vi "test Scheduled Loopback Value Overflow.vi"(8 "error in":errorcluster, 11 "TestCase in":refnum<class "Octal Loopback.lvclass">) -> (0 "error out":errorcluster, 3 "TestCase out":refnum<class "Octal Loopback.lvclass">)   [LabVIEW 2020, in "Octal Loopback.lvclass"]
uses:
  Octal Loopback.lvclass
  C:/Program Files (x86)/National Instruments/LabVIEW 2020/vi.lib/NI/VeriStand Custom Device Testing Tools/VeriStandTestCase/VeriStandTestCase.lvclass
  <vilib>/numeric/Random Number (Range) U64.vi
  <vilib>/numeric/sub_Random U32.vi
  <vilib>/NI VeriStand/Execution/Workspace/NI VeriStand - Set Multiple Channel Values.vi
  <vilib>/addons/_JKI Toolkits/VI Tester/TestCase.llb/TestCase.lvclass
  <vilib>/NI VeriStand/Execution/Workspace/NI_VS Workspace ExecutionAPI.lvlib
  <vilib>/NI/VeriStand Custom Device Testing Tools/VeriStandTestUtilities/VeriStandTestUtilities.lvlib
  C:/Program Files (x86)/National Instruments/LabVIEW 2020/vi.lib/addons/_JKI Toolkits/VI Tester/TestCase.llb/TestCase.lvclass
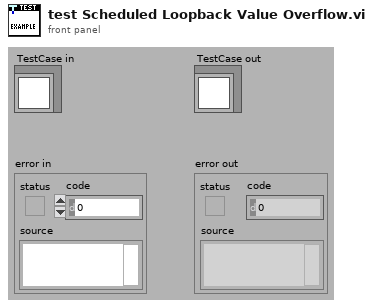
[diagram p1: front panel]
types:
  T1 = typedef "NI_VS Workspace ExecutionAPI.lvlib/WorkspaceAPI.ctl" = refnum<k24>
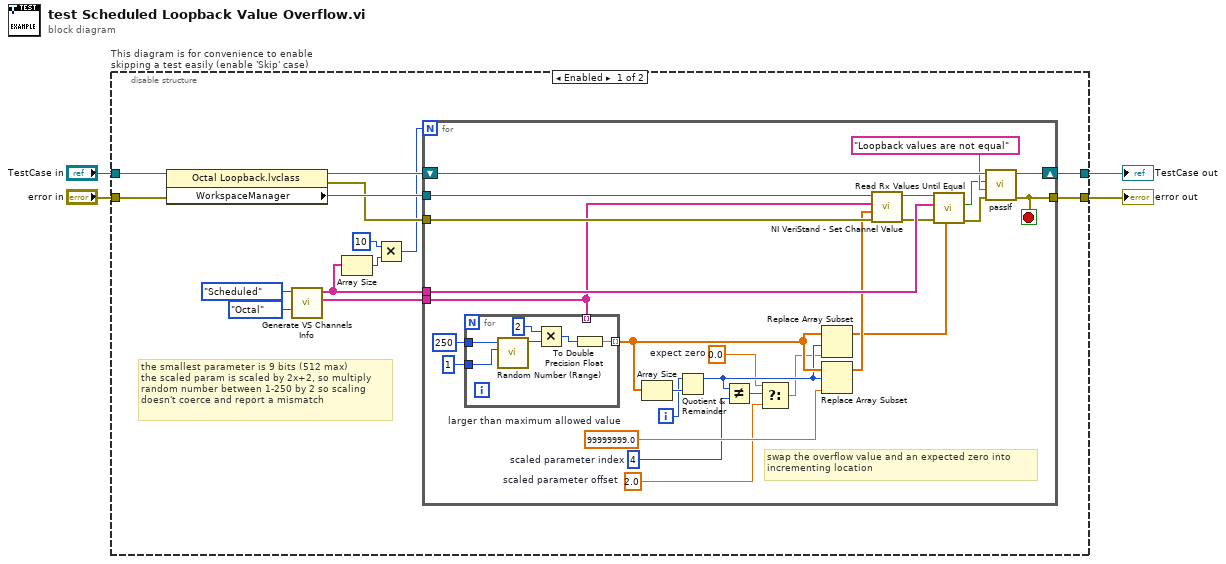
[diagram p0: block diagram]
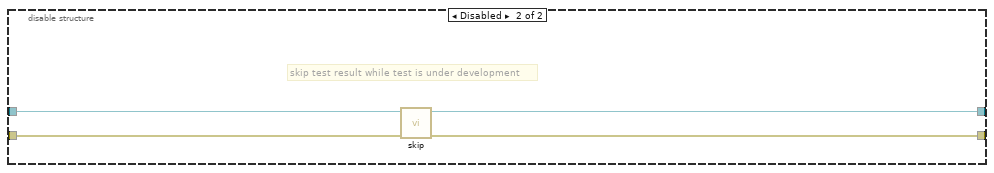
[diagram p2: hidden frame]
diagram:
  n1 = disable-structure "This diagram is for convenience to enable skipping a test easily (enable 'Skip' case)" shown="Enabled" {
    disable-tunnel: "TestCase in" -> [w15 w54]
    disable-tunnel: [w13 w52] -> w1
    disable-tunnel: [w12 w53] -> w3
    disable-tunnel: "error in" -> [w14 w51]
    frame Enabled {
      # "the smallest parameter is 9 bits (512 max)\nthe scaled param is scaled by 2x+2, so multiply \nrandom number between 1-250 by 2 so scaling\ndoesn't coerce and report a mismatch"
      n2 = property class="Octal Loopback.lvclass"(reference=w15, error in=w14) -> (reference out=w16:refnum<class "Octal Loopback.lvclass">, error out=w17:errorcluster, "WorkspaceManager"=w18:T1)
      n3 = call "Generate VS Channels Info.vi"("Label Format (Decimal)"=enum16{"Decimal", "Octal"}."Octal", "Transfer Type"=enum16{"Acyclic", "Scheduled"}."Scheduled") -> ("Tx Channels Array"=w11:string[], "Rx Channels Array"=w10:string[])  [unwired: 5 in, 3 out]
      n4 = Array Size(array=w10) -> (size(s)=w9:i32)
      n5 = Multiply(x=10, y=w9) -> (x*y=w7:i32)
      n6 = for {
        N: w7 -> [_]
        tunnel: w10 -> [w37]
        tunnel: w18 -> [w31]
        tunnel: w17 -> [w36]
        tunnel: w11 -> [w30]
        shift-right: [w43] -> w13
        shift-left: w16 -> [w44]
        tunnel: [w42] -> w12
        i -> [w25]
        stop <- w42 stop-if-true
        w20 = 2.0  # scaled parameter offset
        w23 = 4  # scaled parameter index
        w21 = 0.0  # expect zero
        w38 = 99999999.0  # larger than maximum allowed value
        # "swap the overflow value and an expected zero into \nincrementing location"
        n7 = for {
          tunnel: [w49] -> w26 mode=indexing
          tunnel: u64 250 ("upper bound (100)") -> [w48]
          tunnel: u64 1 ("upper bound (100)") -> [w47]
          tunnel: w30 -> [_] mode=indexing
          n8 = call-poly <vilib>:"Random Number (Range).vi"("lower bound (0)"=w47, "upper bound (100)"=w48) -> ("number"=w50:u64)  [unwired: 9 in]
          n9 = Multiply(x=u64 2, y=w50) -> (x*y=w46:u64)
          n10 = To Double Precision Float(number=w46) -> (double precision float=w49:dbl)
        }
        n11 = Array Size(array=w26) -> (size(s)=w27:i32)
        n12 = Quotient & Remainder(x=w25, y=w27) -> (x-y*floor(x/y)=w24:i32)  [unwired: 1 out]
        n13 = Not Equal?(x=w24, y=w23) -> (x != y?=w22:bool)
        n14 = Select(t=w21, s=w22, f=w20) -> (s? t:f=w19:dbl)
        n15 = Replace Array Subset(array=w26, new element=w19, index=w24) -> (w28:dbl[])
        n16 = Replace Array Subset(array=w26, new element=w38, index=w24) -> (w29:dbl[])
        n17 = call-poly <vilib>:"NI VeriStand - Set Channel Value.vi"("error in (no error)"=w36, "Values"=w29, "Channels"=w30, "WorkspaceManager in"=w31) -> ("error out"=w35:errorcluster, "WorkspaceManager out"=w32:T1)  [unwired: 6 in]
        n18 = call <vilib>:"Read Rx Values Until Equal.vi"("expected values"=w28, "error in"=w35, "Rx aliases"=w37, "workspace manager in"=w32) -> ("error out"=w34:errorcluster, "values equal expected"=w33:bool)  [unwired: 5 in, 1 out]
        n19 = call-dynamic "passIf.vi"("error in (no error)"=w34, "message (\"\")"="Loopback values are not equal" ("message (\"\")"), "pass"=w33, "TestCase in"=w44) -> ("error out"=w42:errorcluster, "TestCase out"=w43:refnum<class "Octal Loopback.lvclass">)  [unwired: 6 in]
      }
    }
    frame Disabled {
      # "skip test result while test is under development"
      n20 = call <vilib>:"skip.vi"("error in (no error)"=w51, "TestCase in"=w54) -> ("error out"=w53:errorcluster, "TestCase out"=w52:refnum<class "Octal Loopback.lvclass">)  [unwired: 8 in]
    }
  }
  "error out" <- w3
  "TestCase out" <- w1
